vi "check internet access (http).vi"(8 "error in (no error)":errorcluster) -> (0 "error out":errorcluster, 3 "Internet OK":bool)   [LabVIEW 2016]
uses:
  <vilib>/httpClient/LabVIEWHTTPClient.lvlib
panel:
  # "check Internet access (http)"
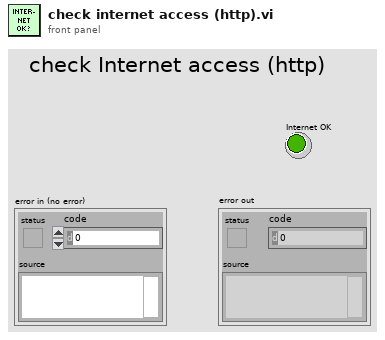
[diagram p1: front panel]
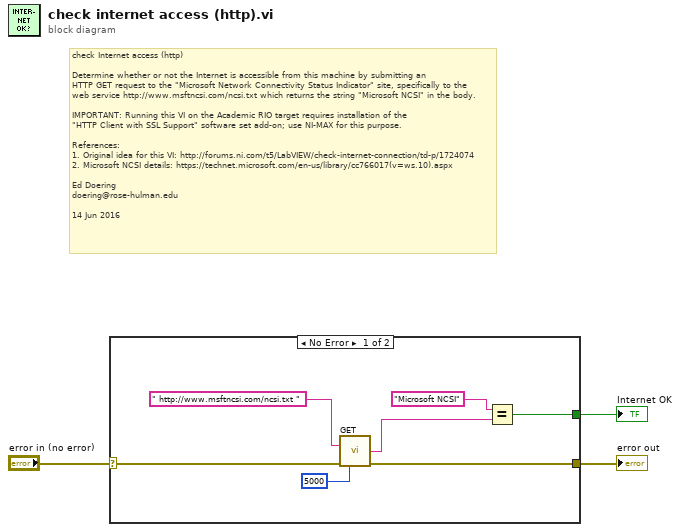
[diagram p0: block diagram]
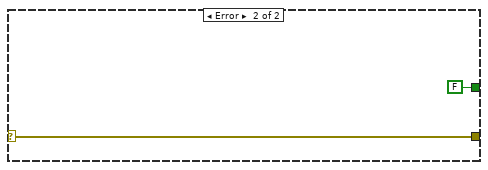
[diagram p2: hidden frame]
diagram:
  # "check Internet access (http)\n\nDetermine whether or not the Internet is accessible from this machine by submitting an\nHTTP GET request to the \"Microsoft Network Connectivity Status Indicator\" site, specifically to the\nweb service http://www.msftncsi.com/ncsi.txt which returns the string \"Microsoft NCSI\" in the body.\n\nIMPORTANT: Running this VI on the Academic RIO target requires installation of the\n\"HTTP Client with SSL Support\" software set add-on; use NI-MAX for this purpose.\n\nReferences:\n1. Original idea for this VI: http://forums.ni.com/t5/LabVIEW/check-internet-connection/td-p/1724074  \n2. Microsoft NCSI details: https://technet.microsoft.com/en-us/library/cc766017(v=ws.10).aspx  \n\nEd Doering\ndoering@rose-hulman.edu\n\n14 Jun 2016"
  n1 = case shown="No Error" "error in (no error)" {
    selector: "error in (no error)" -> [w4 w11]
    tunnel: [w7 FALSE] -> w3
    tunnel: [w6 w11] -> w2
    frame No Error {
      n2 = call <vilib>:"GET.vi"("url"=" http://www.msftncsi.com/ncsi.txt " ("address"), "error in (no error)"=w4, "timeout (10000)"=5000) -> ("body"=w8:string, "error out"=w6:errorcluster)  [unwired: 9 in, 2 out]
      n3 = Equal?(x="Microsoft NCSI", y=w8) -> (x = y?=w7:bool)
    }
    frame Error {
    }
  }
  "Internet OK" <- w3
  "error out" <- w2
